vi "S&E Alarm DigitalString.vi"(2 "Elevated priority":bool, 7 "Content":variant, 9 "error in":errorcluster) -> (8 "format string":string, 10 "error out":errorcluster)   [LabVIEW 2011]
uses:
  reate/S&E Digital Alarm Type.ctl
  GUI/Status Indikator Helper.ctl
  Measurments Handling/Status Digitalish.ctl
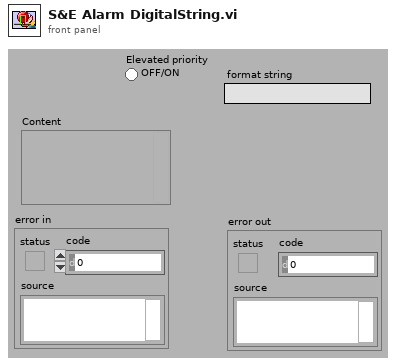
[diagram p1: front panel]
types:
  T1 = typedef "S&E Digital Alarm Type.ctl" = cluster{"Alarm":bool, "Enum":T2, "Value":T3, "Source name":string, "Status text":string}
  T2 = typedef "Status Indikator Helper.ctl" = enum16{"Norm", "L", "H", "LL", "HH", "Value", "Technical"}
  T3 = typedef "Status Digitalish.ctl" = enum16{"NA", "False", "True"}
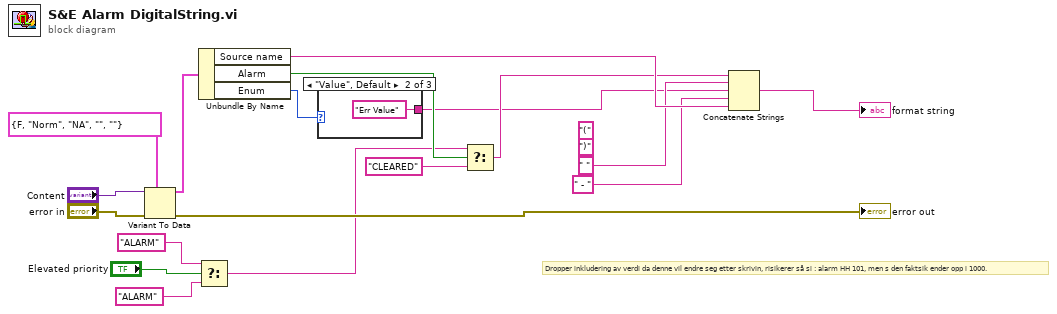
[diagram p0: block diagram]
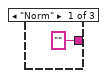
[diagram p2: hidden frame]
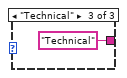
[diagram p3: hidden frame]
diagram:
  (unwired) ")" ("string")
  (unwired) "(" ("string")
  # "Dropper inkludering av verdi da denne vil endre seg etter skrivin, risikerer så si : alarm HH 101, men s den faktsik ender opp i 1000."
  n1 = Variant To Data(error in="error in", type=T1 {"Alarm"=FALSE, "Enum"=enum."Norm", "Value"=enum."NA", "Source name"="", "Status text"=""} ("S&E Alarm"), Variant="Content") -> (data=w14:T1, error out=→"error out":errorcluster)
  n2 = Unbundle By Name(w14) -> ("Source name"=w10:string, "Alarm"=w9:bool, "Enum"=w6:T2)
  n3 = Select(t="ALARM" ("string"), s="Elevated priority", f="ALARM") -> (s? t:f=w8:string)
  n4 = case shown="\"Value\", Default" w6 {
    tunnel: ["" ("string") "Err Value" ("string") "Technical" ("string")] -> w2
    frame "Norm" {
    }
    frame "Value", Default {
    }
    frame "Technical" {
    }
  }
  n5 = Select(t=w8, s=w9, f="CLEARED") -> (s? t:f=w4:string)
  n6 = Concatenate Strings(w4, " " ("string"), w2, " - " ("string"), w10) -> (→"format string":string)
